vi "To Origin File XYdYdX.vi"(4 "Y":dbl[](array[numeric]), 6 "dYdX":dbl[](array[numeric]), 8 "X":dbl[](array[numeric]), 10 "Postfix":string, 11 "Prefix":string) -> (3 "Text":string)   [LabVIEW 2014]
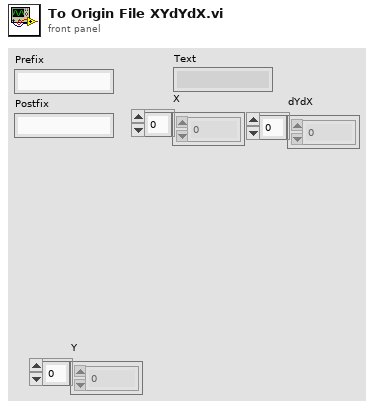
[diagram p1: front panel]
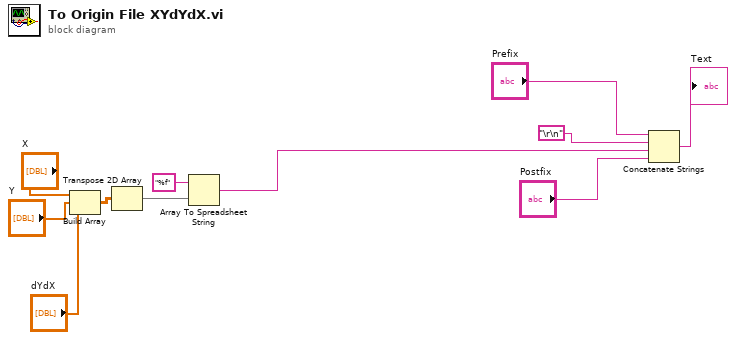
[diagram p0: block diagram]
diagram:
  n1 = Build Array("X", "Y", "dYdX") -> (w9:dbl[][])
  n2 = Transpose 2D Array(2D array=w9) -> (transposed array=w10:dbl[][])
  n3 = Array To Spreadsheet String(array=w10, 3:"%f" ("format string")) -> (spreadsheet string=w4:string)  [unwired: 1 in]
  n4 = Concatenate Strings("Prefix", "\r\n", w4, "Postfix") -> (→"Text":string)
